vi "Write Automation.vi"(8 "error in (no error)":errorcluster, 10 "Automation":refnum<user-event>, 11 "Engine in":refnum<class "Engine.lvclass">) -> (0 "error out":errorcluster, 3 "Engine out":refnum<class "Engine.lvclass">)   [LabVIEW 2019, in "Engine.lvlib" / "Engine.lvclass"]
uses:
  Project/Engine.lvclass
  Project/Engine.lvclass/Engine.ctl
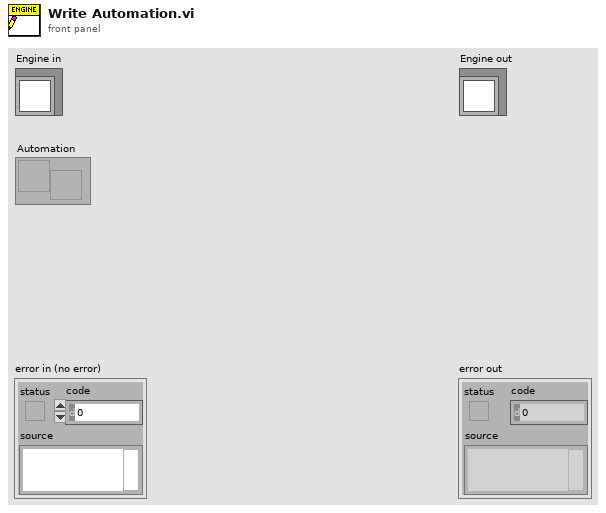
[diagram p1: front panel]
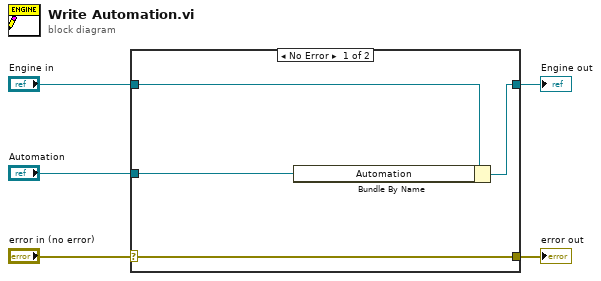
[diagram p0: block diagram]
diagram:
  n1 = case shown="No Error" "error in (no error)" {
    selector: "error in (no error)" -> [w9 w10]
    tunnel: [w9 w10] -> w4
    tunnel: [w7 w11] -> w2
    tunnel: "Engine in" -> [w8 w11]
    tunnel: "Automation" -> [w6 _]
    frame No Error {
      n2 = Bundle By Name(cluster=w8, "Automation"=w6) -> (w7:refnum<class "Engine.lvclass">)
    }
    frame Error {
    }
  }
  "error out" <- w4
  "Engine out" <- w2
